vi "Excel Write Profile.vi"(8 "Error In":errorcluster, 10 "Profile":string[][](array[string]), 11 "Cells Ref In":refnum<k7>) -> (0 "Error Out":errorcluster, 3 "Cells Ref Out":refnum<k7>)   [LabVIEW 2013]
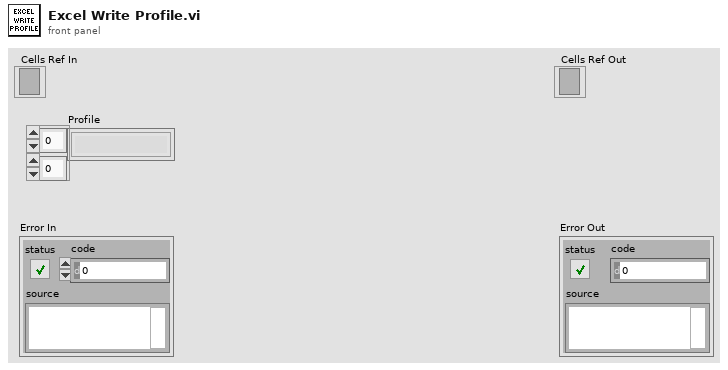
[diagram p1: front panel]
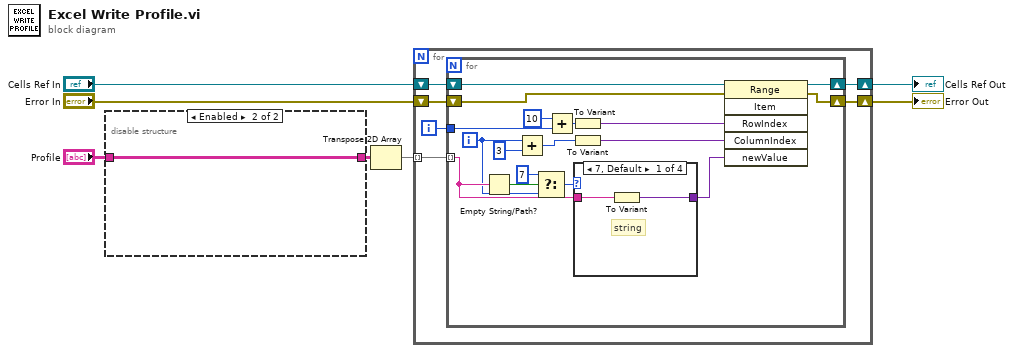
[diagram p0: block diagram]
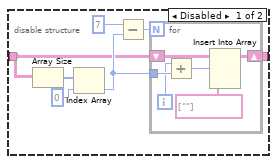
[diagram p2: hidden frame]
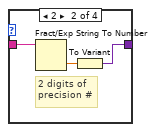
[diagram p3: hidden frame]
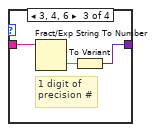
[diagram p4: hidden frame]
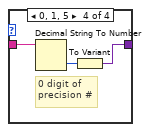
[diagram p5: hidden frame]
diagram:
  n1 = disable-structure shown="Enabled" {
    disable-tunnel: [w14 w21] -> w3
    disable-tunnel: "Profile" -> [w8 w21]
    frame Disabled {
      n2 = Array Size(array=w8) -> (size(s)=w9:i32[])
      n3 = Index Array(array=w9, index=0) -> (element=w13:i32)
      n4 = Subtract(x=7 ("y"), y=w13) -> (x-y=w12:i32)
      n5 = for {
        N: w12 -> [_]
        shift-right: [w18] -> w14
        shift-left: w8 -> [w19]
        tunnel: w13 -> [w16]
        i -> [w15]
        n6 = Add(x=w15, y=w16) -> (x+y=w17:i32)
        n7 = Insert Into Array(array=w19, index (row)=w17, new element=string[] [""]) -> (w18:string[][])  [unwired: 1 in]
      }
    }
    frame Enabled {
    }
  }
  n8 = Transpose 2D Array(2D array=w3) -> (transposed array=w2:string[][])
  n9 = for {
    shift-right: [w25] -> w4
    shift-left: "Cells Ref In" -> [w24]
    shift-right: [w26] -> w5
    shift-left: "Error In" -> [w23]
    tunnel: w2 -> [w27] mode=indexing
    i -> [w22]
    n10 = for {
      shift-right: [w43] -> w25
      shift-left: w24 -> [w44]
      shift-right: [w42] -> w26
      shift-left: w23 -> [w41]
      tunnel: w27 -> [w34] mode=indexing
      tunnel: w22 -> [w36]
      i -> [w30]
      n11 = Empty String/Path?(string/path=w34) -> (empty?=w33:bool)
      n12 = Add(x=w30, y=3) -> (x+y=w29:i32)
      n13 = Select(t=7, s=w33, f=w30) -> (s? t:f=w31:i32)
      n14 = Add(x=10, y=w36) -> (x+y=w38:i32)
      n15 = To Variant(anything=w38) -> (Variant=w40:variant)
      n16 = To Variant(anything=w29) -> (Variant=w39:variant)
      n17 = case shown="7, Default" w31 {
        tunnel: w34 -> [w46 w49 w52 w55]
        tunnel: [w45 w47 w50 w53] -> w35
        frame 7, Default {
          # "string"
          n18 = To Variant(anything=w46) -> (Variant=w45:variant)
        }
        frame 2 {
          # "2 digits of\nprecision #"
          n19 = Fract/Exp String To Number(string=w49) -> (number=w48:dbl)  [unwired: 3 in, 1 out]
          n20 = To Variant(anything=w48) -> (Variant=w47:variant)
        }
        frame 3, 4, 6 {
          # "1 digit of\nprecision #"
          n21 = Fract/Exp String To Number(string=w52) -> (number=w51:dbl)  [unwired: 3 in, 1 out]
          n22 = To Variant(anything=w51) -> (Variant=w50:variant)
        }
        frame 0, 1, 5 {
          # "0 digit of\nprecision #"
          n23 = Decimal String To Number(string=w55) -> (number=w54:i32)  [unwired: 2 in, 1 out]
          n24 = To Variant(anything=w54) -> (Variant=w53:variant)
        }
      }
      n25 = invoke class="Range" method="Item"(reference=w44, error in=w41, "RowIndex"=w40, "ColumnIndex"=w39, "newValue"=w35) -> (reference out=w43:refnum<k7>, error out=w42:errorcluster)  [unwired: 1 in, 4 out]
    }
  }
  "Error Out" <- w5
  "Cells Ref Out" <- w4
